vi "BoardToSinglePicture.vi"(8 "error in (no error)":errorcluster, 10 "Board":T1[][](array[typedef]), 11 "BoardDisplay in":refnum<class "BoardDisplay.lvclass">) -> (0 "error out":errorcluster, 2 "BoardVisulalization":picture[][](array[picture]), 3 "BoardDisplay out":refnum<class "BoardDisplay.lvclass">)   [LabVIEW 2015, in "TronviewPresentation.lvlib" / "BoardDisplay.lvclass"]
uses:
  BoardDisplay.lvclass
  TrajectoryBoardField.ctl
  TrajectoryFieldType.ctl
  TronVIEWBotAPI/MovementDirection.ctl
  BoardDisplay.lvclass/BoardDisplay.ctl
  TronVIEWBotAPI/TronVIEWBotAPI.lvlib
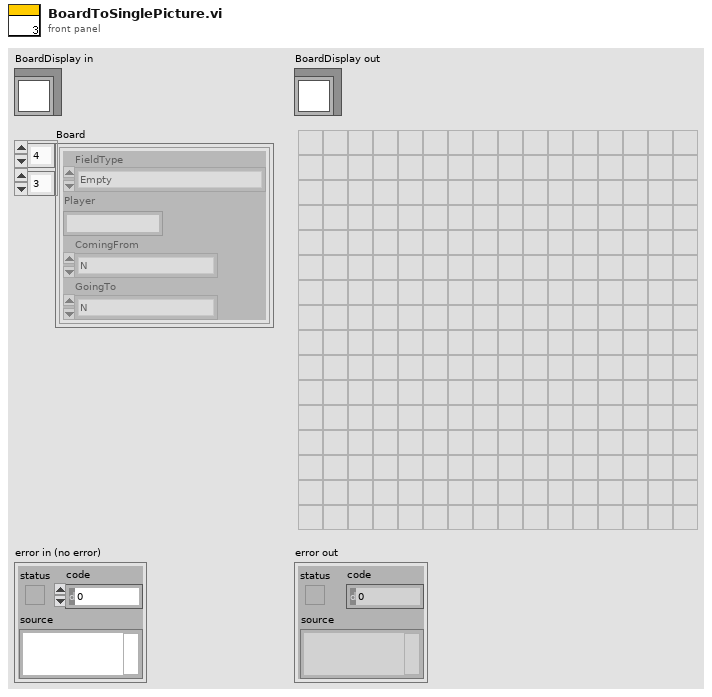
[diagram p1: front panel]
types:
  T1 = typedef "TronviewPresentation.lvlib/BoardDisplay.lvclass/TrajectoryBoardField.ctl" = cluster{"FieldType":T2, "Player":string, "ComingFrom":T3, "GoingTo":T3}
  T2 = typedef "TronviewPresentation.lvlib/BoardDisplay.lvclass/TrajectoryFieldType.ctl" = enum16{"Empty", "Initial", "PlayerWall", "PlayerPosition"}
  T3 = typedef "TronVIEWBotAPI.lvlib/MovementDirection.ctl" = enum16{"N", "S", "W", "E"}
  T4 = typedef "imagedata.ctl" = cluster{"image type":i32, "image depth":i32, "image":u8[], "mask":u8[], "colors":u32[], "Rectangle":cluster{"left":i16, "top":i16, "right":i16, "bottom":i16}}
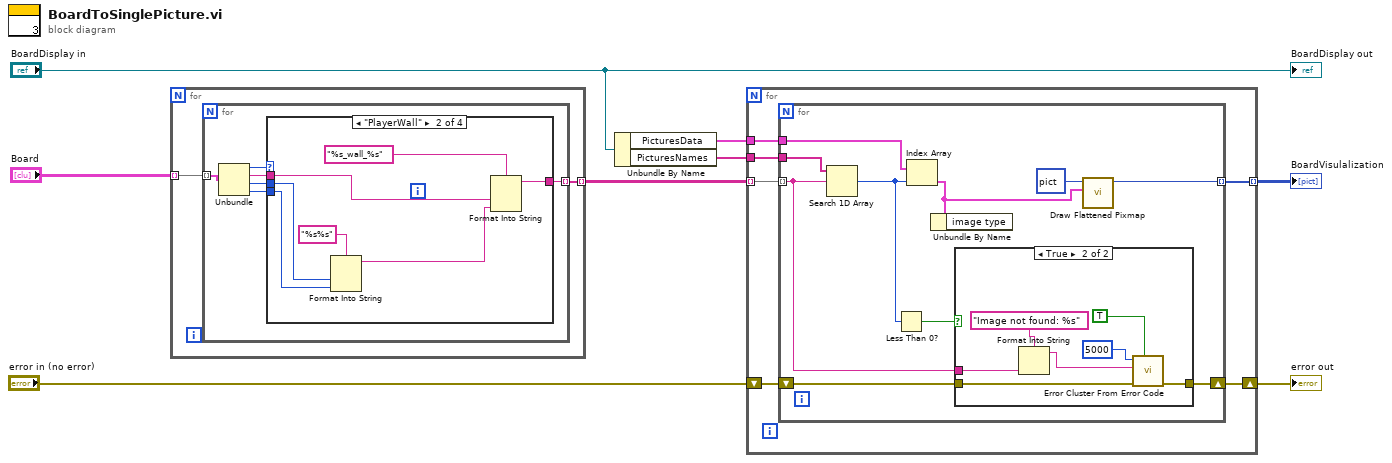
[diagram p0: block diagram]
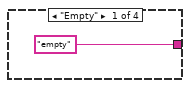
[diagram p2: hidden frame]
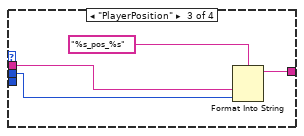
[diagram p3: hidden frame]
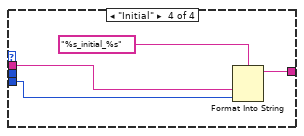
[diagram p4: hidden frame]
diagram:
  n1 = for {
    tunnel: [w10] -> w8 mode=indexing
    tunnel: "Board" -> [w9] mode=indexing
    n2 = for {
      tunnel: [w16] -> w10 mode=indexing
      tunnel: w9 -> [w14] mode=indexing
      n3 = Unbundle(w14) -> ("FieldType"=w13:T2, "Player"=w15:string, "ComingFrom"=w12:T3, "GoingTo"=w11:T3)
      n4 = case shown="\"PlayerWall\"" w13 {
        tunnel: ["empty" w22 w26 w30] -> w16
        tunnel: w15 -> [_ w23 w27 w31]
        tunnel: w12 -> [_ w19 w25 _]
        tunnel: w11 -> [_ w20 _ w29]
        frame "Empty" {
        }
        frame "PlayerWall" {
          n5 = Format Into String(format string="%s%s", w19, w20) -> (resulting string=w18:string)  [unwired: 2 in, 1 out]
          n6 = Format Into String(format string="%s_wall_%s", w23, w18) -> (resulting string=w22:string)  [unwired: 2 in, 1 out]
        }
        frame "PlayerPosition" {
          n7 = Format Into String(format string="%s_pos_%s", w27, w25) -> (resulting string=w26:string)  [unwired: 2 in, 1 out]
        }
        frame "Initial" {
          n8 = Format Into String(format string="%s_initial_%s", w31, w29) -> (resulting string=w30:string)  [unwired: 2 in, 1 out]
        }
      }
    }
  }
  n9 = Unbundle By Name("BoardDisplay in") -> ("PicturesData"=w4:T4[], "PicturesNames"=w5:string[])
  n10 = for {
    tunnel: w8 -> [w38] mode=indexing
    tunnel: w5 -> [w37]
    tunnel: w4 -> [w36]
    tunnel: [w35] -> w3 mode=indexing
    shift-right: [w34] -> w1
    shift-left: "error in (no error)" -> [w33]
    n11 = for {
      tunnel: w38 -> [w42] mode=indexing
      tunnel: w37 -> [w48]
      tunnel: w36 -> [w47]
      tunnel: [w40] -> w35 mode=indexing
      shift-right: [w44] -> w34
      shift-left: w33 -> [w46]
      n12 = Search 1D Array(1D array=w48, element=w42) -> (index of element=w45:i32)  [unwired: 1 in]
      n13 = Less Than 0?(x=w45) -> (x < 0?=w43:bool)
      n14 = Index Array(array=w47, index=w45) -> (element=w39:T4)
      n15 = Unbundle By Name(w39) -> ()  [unwired: 1 out]
      n16 = case shown="True" w43 {
        tunnel: w46 -> [w49 w56]
        tunnel: [w49 w55] -> w44
        tunnel: w42 -> [_ w52]
        frame False {
        }
        frame True {
          n17 = Format Into String(format string="Image not found: %s" ("error message (\"\")"), w52) -> (resulting string=w51:string)  [unwired: 2 in, 1 out]
          n18 = call <vilib>:"Error Cluster From Error Code.vi"("show call chain? (False)"=TRUE, "error in (no error)"=w56, "error message (\"\")"=w51, "error code (0)"=5000) -> ("error out"=w55:errorcluster)  [unwired: 5 in]
        }
      }
      n19 = call <vilib>:"Draw Flattened Pixmap.vi"("image data"=w39, "picture"=picture data[5B]) -> ("new picture"=w40:picture)  [unwired: 7 in]
    }
  }
  "error out" <- w1
  "BoardVisulalization" <- w3
  "BoardDisplay out" <- "BoardDisplay in"
